vi "MTMount_getSample_TopEndChiller.vi"(8 "error in (no error)":errorcluster, 11 "Top_End_Chiller_Ctl":T1) -> (0 "error out":errorcluster, 2 "function return":i32, 3 "Top_End_Chiller_Ctl out":T1)   [LabVIEW 2018, in "SALLV_MTMount.lvlib"]
doc: "int MTMount_shm_getSample_Top_End_ChillerLV(MTMount_Top_End_ChillerLV *Top_End_Chiller_Ctl );"
uses:
  SALLV_MTMount.lvlib
  DataTypes/Top_End_Chiller.ctl
  SALLV_MTMount.so
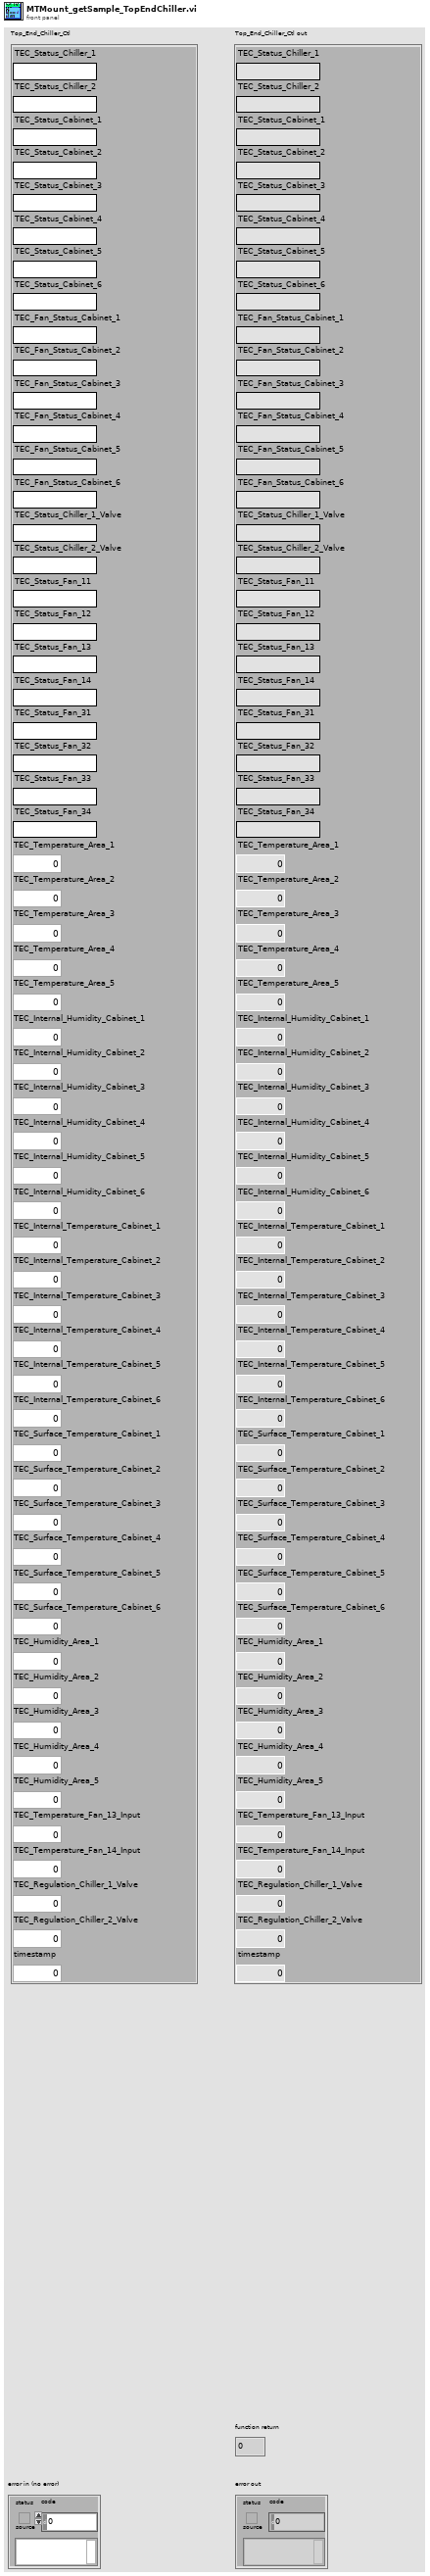
[diagram p1: front panel]
types:
  T1 = typedef "SALLV_MTMount.lvlib/Top_End_Chiller.ctl" = cluster{"TEC_Status_Chiller_1":string, "TEC_Status_Chiller_2":string, "TEC_Status_Cabinet_1":string, "TEC_Status_Cabinet_2":string, "TEC_Status_Cabinet_3":string, "TEC_Status_Cabinet_4":string, "TEC_Status_Cabinet_5":string, "TEC_Status_Cabinet_6":string, "TEC_Fan_Status_Cabinet_1":string, "TEC_Fan_Status_Cabinet_2":string, "TEC_Fan_Status_Cabinet_3":string, "TEC_Fan_Status_Cabinet_4":string, "TEC_Fan_Status_Cabinet_5":string, "TEC_Fan_Status_Cabinet_6":string, "TEC_Status_Chiller_1_Valve":string, "TEC_Status_Chiller_2_Valve":string, "TEC_Status_Fan_11":string, "TEC_Status_Fan_12":string, "TEC_Status_Fan_13":string, "TEC_Status_Fan_14":string, "TEC_Status_Fan_31":string, "TEC_Status_Fan_32":string, "TEC_Status_Fan_33":string, "TEC_Status_Fan_34":string, "TEC_Temperature_Area_1":dbl, "TEC_Temperature_Area_2":dbl, "TEC_Temperature_Area_3":dbl, "TEC_Temperature_Area_4":dbl, "TEC_Temperature_Area_5":dbl, "TEC_Internal_Humidity_Cabinet_1":dbl, "TEC_Internal_Humidity_Cabinet_2":dbl, "TEC_Internal_Humidity_Cabinet_3":dbl, "TEC_Internal_Humidity_Cabinet_4":dbl, "TEC_Internal_Humidity_Cabinet_5":dbl, "TEC_Internal_Humidity_Cabinet_6":dbl, "TEC_Internal_Temperature_Cabinet_1":dbl, "TEC_Internal_Temperature_Cabinet_2":dbl, "TEC_Internal_Temperature_Cabinet_3":dbl, "TEC_Internal_Temperature_Cabinet_4":dbl, "TEC_Internal_Temperature_Cabinet_5":dbl, "TEC_Internal_Temperature_Cabinet_6":dbl, "TEC_Surface_Temperature_Cabinet_1":dbl, "TEC_Surface_Temperature_Cabinet_2":dbl, "TEC_Surface_Temperature_Cabinet_3":dbl, "TEC_Surface_Temperature_Cabinet_4":dbl, "TEC_Surface_Temperature_Cabinet_5":dbl, "TEC_Surface_Temperature_Cabinet_6":dbl, "TEC_Humidity_Area_1":dbl, "TEC_Humidity_Area_2":dbl, "TEC_Humidity_Area_3":dbl, "TEC_Humidity_Area_4":dbl, "TEC_Humidity_Area_5":dbl, "TEC_Temperature_Fan_13_Input":dbl, "TEC_Temperature_Fan_14_Input":dbl, "TEC_Regulation_Chiller_1_Valve":dbl, "TEC_Regulation_Chiller_2_Valve":dbl, "timestamp":dbl}
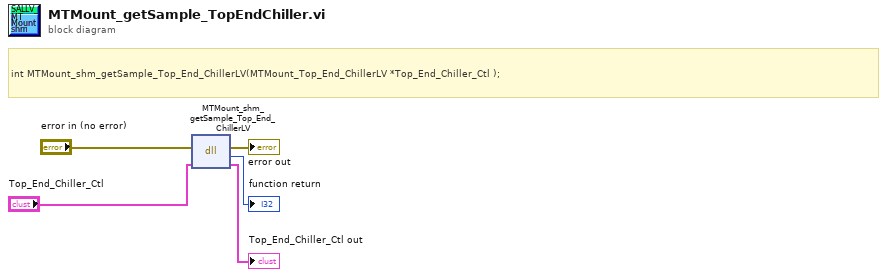
[diagram p0: block diagram]
diagram:
  # "int MTMount_shm_getSample_Top_End_ChillerLV(MTMount_Top_End_ChillerLV *Top_End_Chiller_Ctl );"
  n1 = dll-call lib="home/ttsai/Document/salApiMTMount/SALLV_MTMount/SALLV_MTMount.*" fn="MTMount_shm_getSample_Top_End_ChillerLV"(error in="error in (no error)", "Top_End_Chiller_Ctl"="Top_End_Chiller_Ctl") -> (error out=→"error out":errorcluster, →"function return":i32, "Top_End_Chiller_Ctl"=→"Top_End_Chiller_Ctl out":T1)  [unwired: 2 in, 1 out]
